vi "ArmControlManager.vi"(0 "Arm Rotate Manual Control":dbl, 1 "Arm Extend Manual Control":dbl, 2 "rotate sensor unit conversion (ticks/rad)":dbl, 3 "extend sensor unit coversion (ticks/in)":dbl, 4 "Arm Rotate Motion Profile":T1[](array[typedef]) {"Time (ms)" items=["TrajectoryDuration_0ms"=0, "TrajectoryDuration_5ms"=5, "TrajectoryDuration_10ms"=10, "TrajectoryDuration_20ms"=20, "TrajectoryDuration_30ms"=30, "TrajectoryDuration_40ms"=40, "TrajectoryDuration_50ms"=50, "TrajectoryDuration_100ms"=100]}, 5 "Arm Extend Motion Profile":T1[](array[typedef]) {"Time (ms)" items=["TrajectoryDuration_0ms"=0, "TrajectoryDuration_5ms"=5, "TrajectoryDuration_10ms"=10, "TrajectoryDuration_20ms"=20, "TrajectoryDuration_30ms"=30, "TrajectoryDuration_40ms"=40, "TrajectoryDuration_50ms"=50, "TrajectoryDuration_100ms"=100]}, 8 "Arm Extend Motor DevRef":T4={"DeviceStatus"={"status"=FALSE, "code"=0, "source"=""}, "Type"=enum."PWM", "PWM"={"PWM Channel"=enum."PWM 1", "DeadBand"={"Name"="", "maxPositivePwm"=0, "minPositivePwm"=0, "centerPwm"=0, "maxNegativePwm"=0, "minNegativePwm"=0, "angularRange"=0}}, "CAN"={"Device Number"=0, "SetOutput VI Ref"=variant(enum8{"Percent VBus", "Current", "Speed", "Position", "Voltage"} enum."Percent VBus"), "GetOutput VI Ref"=variant(refnum<k1> refnum), "Enable VI Ref"=variant(dbl 12.0), "Disable VI Ref"=variant(enum8{"Percent VBus", "Speed", "Position", "Slave", "Unchanged / Invalid", "Voltage Compensation", "Current", "Motion Profile"} enum."Percent VBus"), "Data"=variant}, "Invert"=FALSE, "DIO PWM"={"PWM \"Enable\" Channel"=enum."Invalid", "DIOChannel"=enum."Invalid", "PWM Rate"=0.0}}, 9 "New Motion Profile":bool, 10 "Arm Rotate Motor DevRef":T4={"DeviceStatus"={"status"=FALSE, "code"=0, "source"=""}, "Type"=enum."PWM", "PWM"={"PWM Channel"=enum."PWM 1", "DeadBand"={"Name"="", "maxPositivePwm"=0, "minPositivePwm"=0, "centerPwm"=0, "maxNegativePwm"=0, "minNegativePwm"=0, "angularRange"=0}}, "CAN"={"Device Number"=0, "SetOutput VI Ref"=variant(enum8{"Percent VBus", "Current", "Speed", "Position", "Voltage"} enum."Percent VBus"), "GetOutput VI Ref"=variant(refnum<k1> refnum), "Enable VI Ref"=variant(dbl 12.0), "Disable VI Ref"=variant(enum8{"Percent VBus", "Speed", "Position", "Slave", "Unchanged / Invalid", "Voltage Compensation", "Current", "Motion Profile"} enum."Percent VBus"), "Data"=variant}, "Invert"=FALSE, "DIO PWM"={"PWM \"Enable\" Channel"=enum."Invalid", "DIOChannel"=enum."Invalid", "PWM Rate"=0.0}}) -> (14 "Arm Control State":T3)   [LabVIEW 2017]
uses:
  General/MotionProfiling/TypeDefs/TrajectoryPoint.ctl
  <vilib>/Rock Robotics/WPI/ThirdParty/Phoenix-LabVIEW/Motor Controller/Controls/CTRE_Phoenix_MotorControl_TrajectoryPointTimeDur.ctl
  General/MotionProfiling/TypeDefs/MotionProfileControlState.ctl
  <vilib>/Rock Robotics/WPI/MotorControl/WPI_MotorControlDeviceRef.ctl
  <vilib>/Rock Robotics/WPI/MotorControl/WPI_MotorControlType.ctl
  <vilib>/Rock Robotics/SystemInterfaces/DIO/FPGA_DIOPWMChannel.ctl
  <vilib>/Rock Robotics/WPI/PWM/WPI_PWMDeadband.ctl
  <vilib>/Rock Robotics/SystemInterfaces/DIO/FPGA_DIOChannel.ctl
  <vilib>/Rock Robotics/WPI/DriverStation/WPI_DriverStationRobotMode2.ctl
  ArgosLib/Signal Processing/TypeDefs/EdgeDetector_Type.ctl
  <vilib>/Rock Robotics/WPI/ThirdParty/Phoenix-LabVIEW/Motor Controller/Controls/CTRE_Phoenix_MotorControl_ControlMode.ctl
  <vilib>/Rock Robotics/WPI/ThirdParty/Phoenix-LabVIEW/Motor Controller/Get/CTRE_Phoenix_MotorController_GetSelectedSensorData.vi
  <vilib>/Rock Robotics/WPI/ThirdParty/Phoenix-LabVIEW/Motor Controller/Get/CTRE_Phoenix_MotorController_GetClosedLoopData.vi
  <vilib>/Rock Robotics/WPI/ThirdParty/Phoenix-LabVIEW/Motor Controller/Get/CTRE_Phoenix_MotorController_GetVoltage.vi
  ArgosLib/ArgosLib.lvlib
panel:
  in  "Tab Control":enum32{"I/O", "Calibration", "Status"}(tab)
  in  "ExtendErrorThresh (in)":dbl=3.0
  in  "RotateErrorThresh (rad)":dbl=0.1745
  in  "ClearMotionProfile":bool
  in  "StallDetectTime(ms)":u32=200
  out "Max Extend Speed (Sensor Units per 100 ms)":i32
  out "Max Rotate Speed (Sensor Units per 100 ms)":i32
  in  "Reset Rotate Max":bool
  in  "Reset Extend Max":bool
  in  "Reset Extend Sensor":bool
  in  "Reset Rotate Sensor":bool
  in  "Extend Position (in)":dbl=-44.0
  in  "Rotate Position (rad)":dbl=1.57
  out "Rotate":T9
  out "Extension":T9
  out "Rotate":T10
  out "Extension":T10
  out "ExtendFaults":T11
  out "RotateFaults":T11
  out "Arm Tracking":cluster{dbl[], dbl[]}[](graph)
  out "ArmRotateV":dbl(graph)
  out "ArmExtensionV":dbl(graph)
  out "ArmExtension":T10(graph)
  out "ArmRotation":T10(graph)
  # "10 degrees or 3 inches\nerror for 200ms will\ncancel motion"
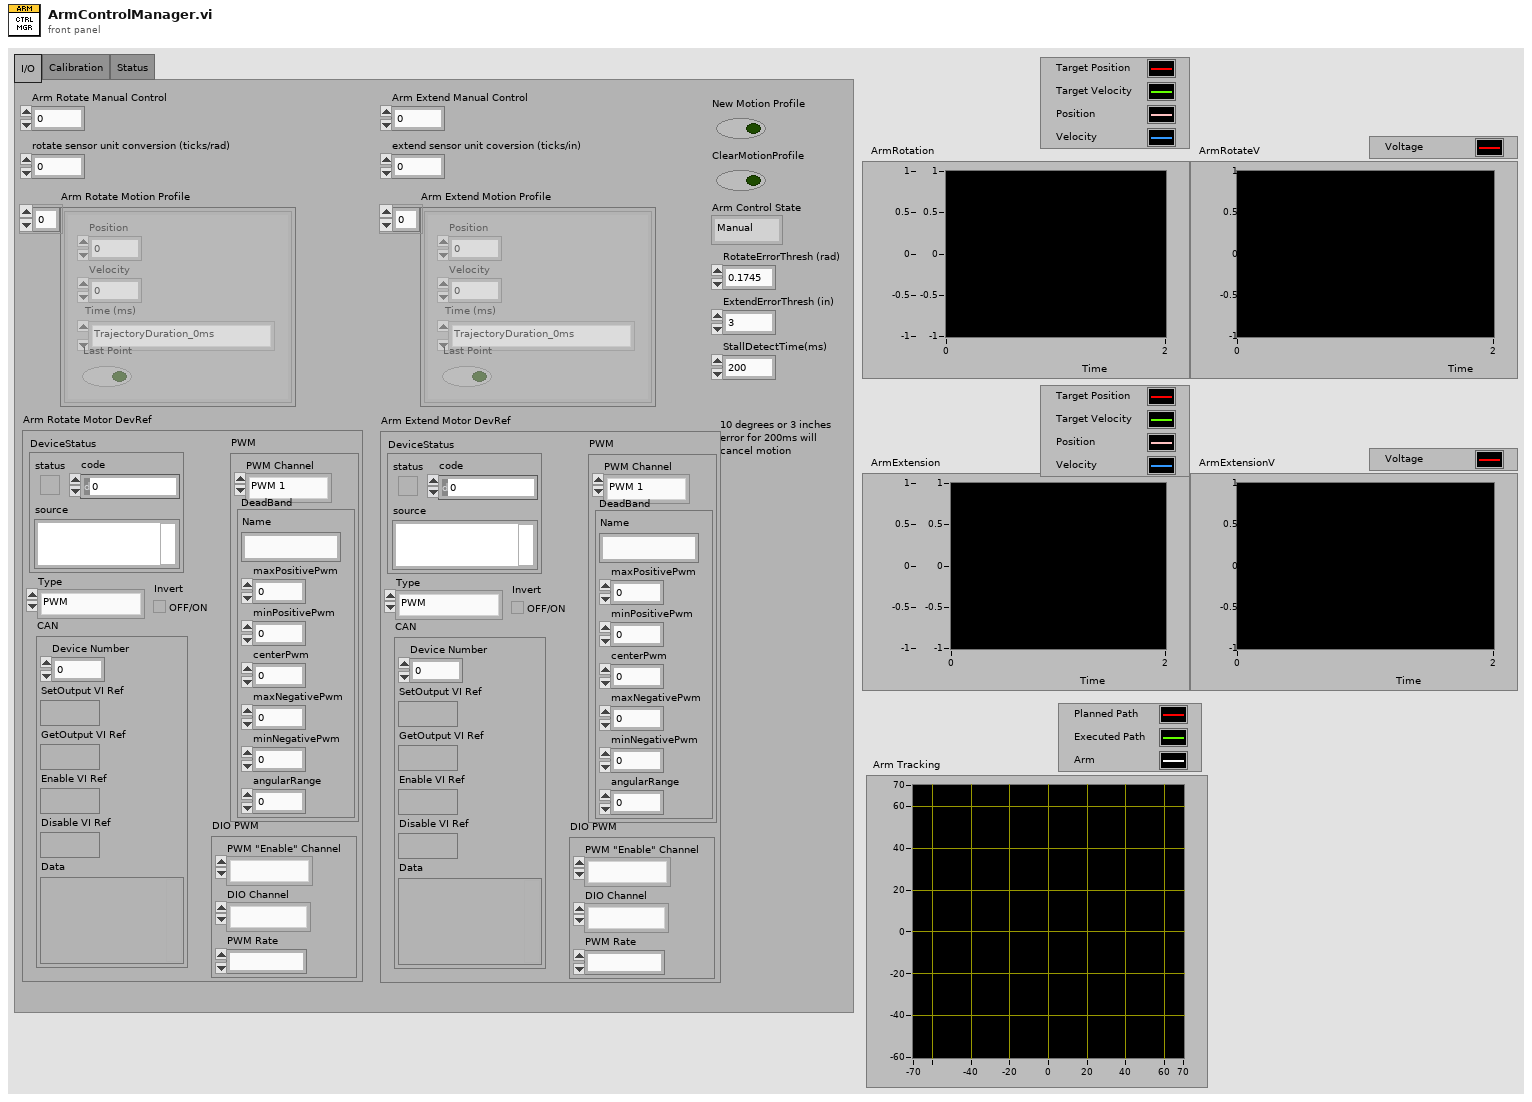
[diagram p1: front panel]
types:
  T1 = typedef "TrajectoryPoint.ctl" = cluster{"Position ":dbl, "Velocity ":dbl, "Time (ms)":T2, "Last Point":bool}
  T2 = typedef "CTRE_Phoenix_MotorControl_TrajectoryPointTimeDur.ctl" = i32
  T3 = typedef "MotionProfileControlState.ctl" = enum16{"Manual", "Auto_Idle", "Auto_Run"}
  T4 = typedef "WPI_MotorControlDeviceRef.ctl" = cluster{"DeviceStatus":errorcluster, "Type":T5, "PWM":cluster{"PWM Channel":T6, "DeadBand":T7}, "CAN":cluster{"Device Number":u8, "SetOutput VI Ref":variant, "GetOutput VI Ref":variant, "Enable VI Ref":variant, "Disable VI Ref":variant, "Data":variant}, "Invert":bool, "DIO PWM":cluster{"PWM \"Enable\" Channel":T6, "DIOChannel":T8, "PWM Rate":dbl}}
  T5 = typedef "WPI_MotorControlType.ctl" = enum16{"PWM", "CAN", "DIO PWM"}
  T6 = typedef "FPGA_DIOPWMChannel.ctl" = enum8{"PWM 0", "PWM 1", "PWM 2", "PWM 3", "PWM 4", "PWM 5", "PWM 6", "PWM 7", "PWM 8", "PWM 9", "PWM MXP 0", "PWM MXP 1", "PWM MXP 2", "PWM MXP 3", "PWM MXP 4", "PWM MXP 5", "PWM MXP 6", "PWM MXP 7", "PWM MXP 8", "PWM MXP 9", "Invalid"}
  T7 = typedef "WPI_PWMDeadband.ctl" = cluster{"Name":string, "maxPositivePwm":i32, "minPositivePwm":i32, "centerPwm":i32, "maxNegativePwm":i32, "minNegativePwm":i32, "angularRange":u16}
  T8 = typedef "FPGA_DIOChannel.ctl" = enum8{"DIO 0", "DIO 1", "DIO 2", "DIO 3", "DIO 4", "DIO 5", "DIO 6", "DIO 7", "DIO 8", "DIO 9", "DIO MXP 0", "DIO MXP 1", "DIO MXP 2", "DIO MXP 3", "DIO MXP 4", "DIO MXP 5", "DIO MXP 6", "DIO MXP 7", "DIO MXP 8", "DIO MXP 9", "DIO MXP 10", "DIO MXP 11", "DIO MXP 12", "DIO MXP 13", "DIO MXP 14", "DIO MXP 15", "SPI Port CS1", "SPI Port CS2", "SPI Port CS3", "SPI Port MISO", "SPI Port MOSI", "Invalid"}
  T9 = cluster{"Top Buffer Remaining":i32, "Top Buffer Count":i32, "Bottom Buffer Count":i32, "Has Underrun?":bool, "Is Underrun?":bool, "Active Point Valid?":bool, "Is Last?":bool, "Profile Slot Select 0":i32, "Output Enable":i32, "Time Duration (ms)":i32, "Profile Slot Select 1":i32}
  T10 = cluster{"Position (Sensor Units)":i32, "Velocity (Sensor Units per 100 ms)":i32, "Position (Raw Sensor Units)":i32, "Velocity (Raw Sensor Units per 100 ms)":i32}
  T11 = cluster{"Under Voltage":bool, "Forward Limit Switch":bool, "Reverse Limit Switch":bool, "Forward Soft Limit":bool, "Reverse Soft Limit":bool, "Hardware Failure":bool, "Reset During Enable":bool, "Sensor Overflow":bool, "Sensor Out of Phase":bool, "Hardware ESD Reset":bool, "Remote Loss of Signal":bool}
  T12 = typedef "WPI_DriverStationRobotMode2.ctl" = enum16{"Autonomous Disabled", "Autonomous Enabled", "Teleop Disabled", "Teleop Enabled", "Disconnected", "Finish", "Test Disabled", "Test Enabled", "Emergency Stopped"}
  T13 = typedef "ArgosLib.lvlib/EdgeDetector_Type.ctl" = enum16{"RisingEdge", "FallingEdge", "Both"}
  T14 = cluster{"Position (Sensor Units)":i32, "Velocity (Sensor Units per 100 ms)":i32, "Position (Raw Sensor Units)":i32, "Velocity (Raw Sensor Units per 100 ms)":i32}[]
  T15 = typedef "CTRE_Phoenix_MotorControl_ControlMode.ctl" = u16
  T16 = cluster{"Position (Sensor Units)":i32, "Velocity (Sensor Units per 100 ms)":i32, "Position (Raw Sensor Units)":i32, i32}
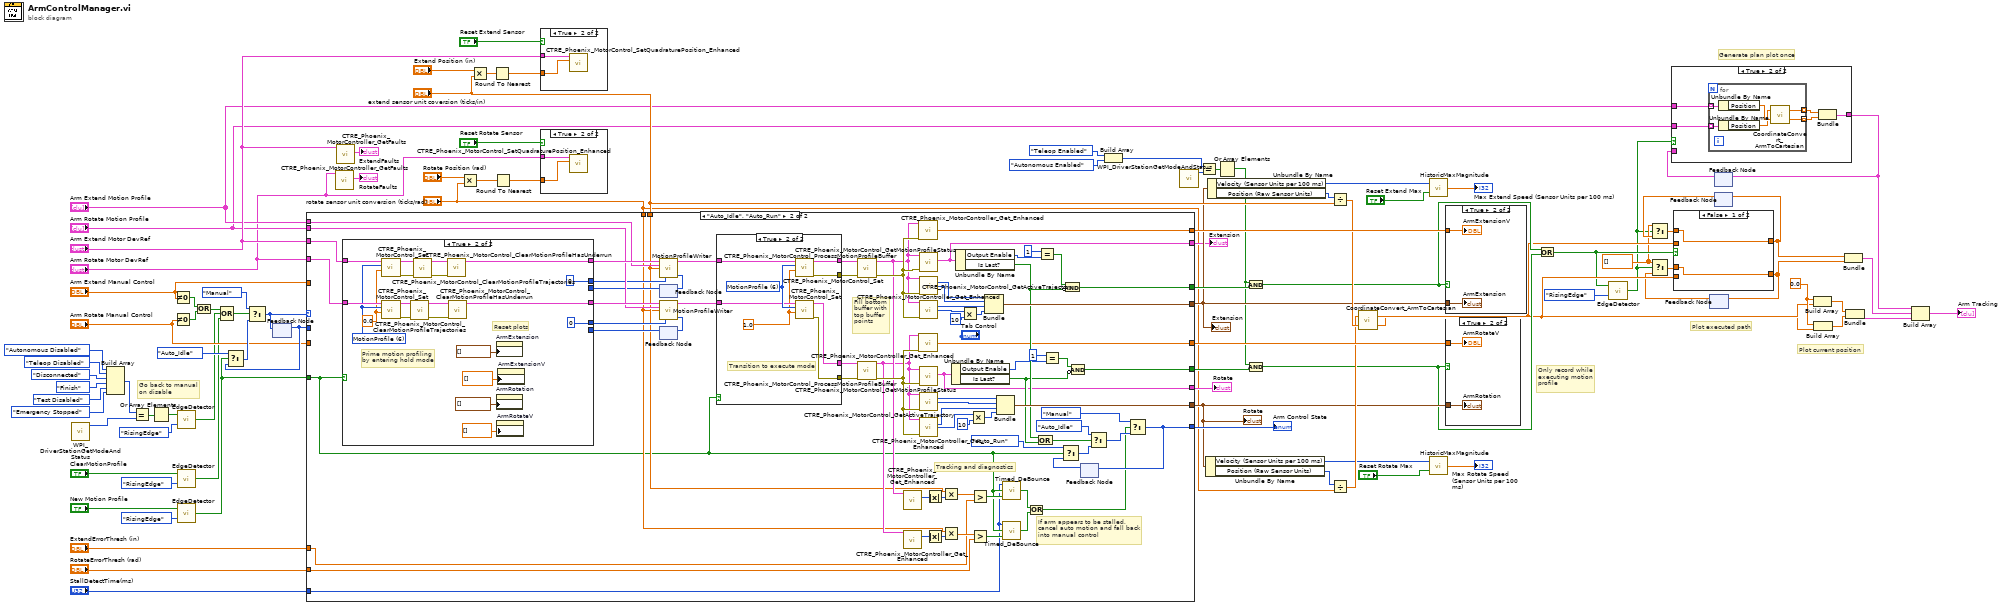
[diagram p0: block diagram]
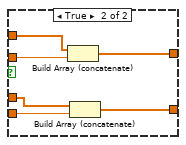
[diagram p3: hidden frame]
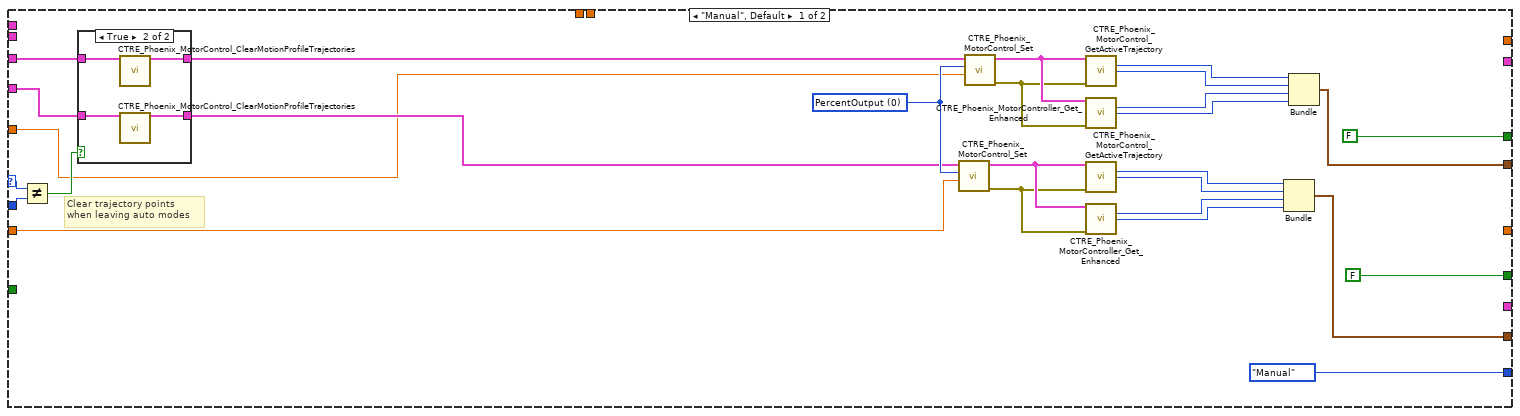
[diagram p8: hidden frame]
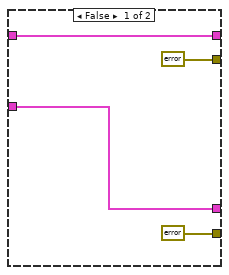
[diagram p10: hidden frame]
diagram:
  w16 = dbl[] [] ("t")
  w53 = 0.0 ("element")
  # "Plot current position"
  # "Plot executed path"
  # "Generate plan plot once"
  # "Go back to manual\non disable"
  # "Only record while\nexecuting motion\nprofile"
  n1 = call <vilib>:"WPI_DriverStationGetModeAndStatus.vi"() -> ("Robot Mode"=w45:T12)  [unwired: 10 in, 1 out]
  n2 = Build Array(WPI_DriverStationRobotMode2."Autonomous Disabled" ("Robot Mode"), WPI_DriverStationRobotMode2."Teleop Disabled" ("Robot Mode"), WPI_DriverStationRobotMode2."Disconnected" ("Robot Mode"), WPI_DriverStationRobotMode2."Finish" ("Robot Mode"), WPI_DriverStationRobotMode2."Test Disabled" ("Robot Mode"), WPI_DriverStationRobotMode2."Emergency Stopped" ("Robot Mode")) -> (w46:T12[])
  n3 = Equal?(x=w46, y=w45) -> (x = y?=w44:bool[])
  n4 = Or Array Elements(Boolean array=w44) -> (logical OR=w43:bool)
  n5 = Not Equal To 0?(x="Arm Extend Manual Control") -> (x != 0?=w95:bool)
  n6 = Not Equal To 0?(x="Arm Rotate Manual Control") -> (x != 0?=w94:bool)
  n7 = call "EdgeDetector.vi"("DetectorType"=EdgeDetector_Type."RisingEdge", "Input"=w43) -> ("Edge"=w40:bool)
  n8 = call "EdgeDetector.vi"("DetectorType"=EdgeDetector_Type."RisingEdge", "Input"="ClearMotionProfile") -> ("Edge"=w41:bool)
  n9 = call "EdgeDetector.vi"("DetectorType"=EdgeDetector_Type."RisingEdge", "Input"="New Motion Profile") -> ("Edge"=w87:bool)
  n10 = Or(x=w95, y=w94) -> (x .or. y?=w72:bool)
  n11 = Compound Arithmetic op=OR(w72, w40, w41) -> (w73:bool)
  n12 = feedback #1() -> (w91:T3)  [unwired: 1 in]
  n13 = Select(t=MotionProfileControlState."Auto_Idle", s=w87, f=w91) -> (s? t:f=w92:T3)
  n14 = Select(t=MotionProfileControlState."Manual" ("Arm Control State"), s=w73, f=w92) -> (s? t:f=w39:T3)
  n15 = feedback-in #1(w39) -> ()
  n16 = case shown="\"Auto_Idle\", \"Auto_Run\"" w39 {
    selector: w39 -> [w120 _]
    tunnel: "Arm Extend Motor DevRef" -> [w117 w203]
    tunnel: "Arm Rotate Motor DevRef" -> [w115 w202]
    tunnel: "Arm Extend Manual Control" -> [w96 _]
    tunnel: "Arm Rotate Manual Control" -> [w121 _]
    tunnel: w91 -> [w119 _]
    tunnel: w87 -> [_ w136]
    tunnel: "Arm Extend Motion Profile" -> [_ w189]
    tunnel: "Arm Rotate Motion Profile" -> [_ w188]
    tunnel: [MotionProfileControlState."Manual" ("Arm Control State") w132] -> w86
    tunnel: [w112 w193] -> w55
    tunnel: [w99 w192] -> w54
    tunnel: [FALSE w173] -> w76
    tunnel: [FALSE w169] -> w79
    tunnel: [_ w160] -> w75
    tunnel: [_ w159] -> w74
    tunnel: "extend sensor unit coversion (ticks/in)" -> [_ w147]
    tunnel: "rotate sensor unit conversion (ticks/rad)" -> [_ w143]
    tunnel: [_ w154] -> w32
    tunnel: [_ w153] -> w31
    tunnel: "ExtendErrorThresh (in)" -> [_ w139]
    tunnel: "RotateErrorThresh (rad)" -> [_ w140]
    tunnel: "StallDetectTime(ms)" -> [_ w135]
    frame "Manual", Default {
      w122 = T15 0 items=["PercentOutput"=0, "Position"=1, "Velocity"=2, "Current"=3, "Follower"=5, "MotionProfile"=6, "MotionMagic"=7, "MotionMagicArc"=8, "MotionProfileArc"=10, "Disabled"=15] ("Control Mode")
      # "Clear trajectory points\nwhen leaving auto modes"
      n17 = Not Equal?(x=w120, y=w119) -> (x != y?=w118:bool)
      n18 = case shown="True" w118 {
        tunnel: w117 -> [w124 w128]
        tunnel: [w124 w127] -> w116
        tunnel: w115 -> [w123 w126]
        tunnel: [w123 w125] -> w114
        frame False {
        }
        frame True {
          n19 = call <vilib>:"CTRE_Phoenix_MotorControl_ClearMotionProfileTrajectories.vi"("PhoenixMotorControlDevRef"=w128) -> ("PhoenixMotorControlDevRef"=w127:T4)  [unwired: 13 in, 1 out]
          n20 = call <vilib>:"CTRE_Phoenix_MotorControl_ClearMotionProfileTrajectories.vi"("PhoenixMotorControlDevRef"=w126) -> ("PhoenixMotorControlDevRef"=w125:T4)  [unwired: 13 in, 1 out]
        }
      }
      n21 = call <vilib>:"CTRE_Phoenix_MotorControl_Set.vi"("Output"=w121, "Control Mode"=w122, "PhoenixMotorControlDevRef"=w114) -> ("error out"=w104:errorcluster, "PhoenixMotorControlDevRef"=w105:T4)  [unwired: 7 in]
      n22 = call <vilib>:"CTRE_Phoenix_MotorControl_Set.vi"("Output"=w96, "Control Mode"=w122, "PhoenixMotorControlDevRef"=w116) -> ("error out"=w110:errorcluster, "PhoenixMotorControlDevRef"=w111:T4)  [unwired: 7 in]
      n23 = call <vilib>:"CTRE_Phoenix_MotorControl_GetActiveTrajectory.vi"("PhoenixMotorControlDevRef"=w111, "error in"=w110) -> ("Position (Sensor Units)"=w109:i32, "Velocity (Sensor Units per 100 ms)"=w108:i32)  [unwired: 9 in, 3 out]
      n24 = call-poly <vilib>:"CTRE_Phoenix_MotorController_Get_Enhanced.vi"("PhoenixMotorControlDevRef"=w111, "error in"=w110) -> ("Position (Raw Sensor Units)"=w107:i32, "Velocity (Raw Sensor Units per 100 ms)"=w106:i32)  [unwired: 10 in, 2 out]
      n25 = call <vilib>:"CTRE_Phoenix_MotorControl_GetActiveTrajectory.vi"("PhoenixMotorControlDevRef"=w105, "error in"=w104) -> ("Position (Sensor Units)"=w103:i32, "Velocity (Sensor Units per 100 ms)"=w102:i32)  [unwired: 9 in, 3 out]
      n26 = call-poly <vilib>:"CTRE_Phoenix_MotorController_Get_Enhanced.vi"("PhoenixMotorControlDevRef"=w105, "error in"=w104) -> ("Position (Raw Sensor Units)"=w101:i32, "Velocity (Raw Sensor Units per 100 ms)"=w100:i32)  [unwired: 10 in, 2 out]
      n27 = Bundle("Position (Sensor Units)"=w103, "Velocity (Sensor Units per 100 ms)"=w102, "Position (Raw Sensor Units)"=w101, "Velocity (Raw Sensor Units per 100 ms)"=w100) -> (w99:T10)  [unwired: 1 in]
      n28 = Bundle("Position (Sensor Units)"=w109, "Velocity (Sensor Units per 100 ms)"=w108, "Position (Raw Sensor Units)"=w107, "Velocity (Raw Sensor Units per 100 ms)"=w106) -> (w112:T10)  [unwired: 1 in]
    }
    frame "Auto_Idle", "Auto_Run" {
      # "If arm appears to be stalled,\ncancel auto motion and fall back\ninto manual control"
      # "Tracking and diagnostics"
      # "Fill bottom\nbuffer with\ntop buffer\npoints"
      n29 = feedback #2() -> (w182:i32)  [unwired: 1 in]
      n30 = feedback #3() -> (w184:i32)  [unwired: 1 in]
      n31 = case shown="True" w136 {
        tunnel: w203 -> [w219 w227]
        tunnel: w202 -> [w218 w224]
        tunnel: [w219 w231] -> w190
        tunnel: [w218 w230] -> w191
        tunnel: [w216 0] -> w187
        tunnel: [w217 0] -> w186
        tunnel: w184 -> [w217 _]
        tunnel: w182 -> [w216 _]
        frame False {
        }
        frame True {
          w222 = 0.0 ("Output")
          w223 = T15 6 items=["PercentOutput"=0, "Position"=1, "Velocity"=2, "Current"=3, "Follower"=5, "MotionProfile"=6, "MotionMagic"=7, "MotionMagicArc"=8, "MotionProfileArc"=10, "Disabled"=15] ("Control Mode")
          # "Prime motion profiling\nby entering hold mode"
          # "Reset plots"
          n32 = call <vilib>:"CTRE_Phoenix_MotorControl_Set.vi"("Output"=w222, "Control Mode"=w223, "PhoenixMotorControlDevRef"=w227) -> ("error out"=w229:errorcluster, "PhoenixMotorControlDevRef"=w228:T4)  [unwired: 7 in]
          n33 = call <vilib>:"CTRE_Phoenix_MotorControl_Set.vi"("Output"=w222, "Control Mode"=w223, "PhoenixMotorControlDevRef"=w224) -> ("error out"=w226:errorcluster, "PhoenixMotorControlDevRef"=w225:T4)  [unwired: 7 in]
          n34 = call <vilib>:"CTRE_Phoenix_MotorControl_ClearMotionProfileTrajectories.vi"("PhoenixMotorControlDevRef"=w225, "error in"=w226) -> ("PhoenixMotorControlDevRef"=w235:T4, "error out"=w234:errorcluster)  [unwired: 12 in]
          n35 = call <vilib>:"CTRE_Phoenix_MotorControl_ClearMotionProfileTrajectories.vi"("PhoenixMotorControlDevRef"=w228, "error in"=w229) -> ("PhoenixMotorControlDevRef"=w233:T4, "error out"=w232:errorcluster)  [unwired: 12 in]
          n36 = call <vilib>:"CTRE_Phoenix_MotorControl_ClearMotionProfileHasUnderrun.vi"("error in"=w232, "PhoenixMotorControlDevRef"=w233) -> ("PhoenixMotorControlDevRef"=w231:T4)  [unwired: 8 in, 1 out]
          n37 = call <vilib>:"CTRE_Phoenix_MotorControl_ClearMotionProfileHasUnderrun.vi"("error in"=w234, "PhoenixMotorControlDevRef"=w235) -> ("PhoenixMotorControlDevRef"=w230:T4)  [unwired: 8 in, 1 out]
          n38 = property on="ArmExtension" class="WFChart (strict)"("History Data"=T14 []) -> ()  [unwired: 2 in, 2 out]
          n39 = property on="ArmRotation" class="WFChart (strict)"("History Data"=T14 []) -> ()  [unwired: 2 in, 2 out]
          n40 = property on="ArmRotateV" class="WFChart (strict)"("History Data"=dbl[] []) -> ()  [unwired: 2 in, 2 out]
          n41 = property on="ArmExtensionV" class="WFChart (strict)"("History Data"=dbl[] []) -> ()  [unwired: 2 in, 2 out]
        }
      }
      n42 = call "MotionProfileWriter.vi"("PhoenixMotorControlDevRef"=w190, "Trajectory Points"=w189, "Sensor unit conversion"=w147, "startIndex"=w187) -> ("PhoenixMotorControlDevRef Out"=w181:T4, "endIndex"=w183:i32)  [unwired: 10 in]
      n43 = feedback-in #2(w183) -> ()
      n44 = call "MotionProfileWriter.vi"("PhoenixMotorControlDevRef"=w191, "Trajectory Points"=w188, "Sensor unit conversion"=w143, "startIndex"=w186) -> ("PhoenixMotorControlDevRef Out"=w179:T4, "endIndex"=w185:i32)  [unwired: 10 in]
      n45 = feedback-in #3(w185) -> ()
      n46 = case shown="True" w136 {
        tunnel: w181 -> [w207 w214]
        tunnel: [w207 w213] -> w180
        tunnel: w179 -> [w206 w212]
        tunnel: [w206 w211] -> w178
        tunnel: [errorcluster {"status"=FALSE, "code"=0, "source"=""} ("error out") w209] -> w152
        tunnel: [errorcluster {"status"=FALSE, "code"=0, "source"=""} ("error out") w208] -> w151
        frame False {
        }
        frame True {
          w210 = 1.0 ("Output")
          w215 = T15 6 items=["PercentOutput"=0, "Position"=1, "Velocity"=2, "Current"=3, "Follower"=5, "MotionProfile"=6, "MotionMagic"=7, "MotionMagicArc"=8, "MotionProfileArc"=10, "Disabled"=15] ("Control Mode")
          # "Transition to execute mode"
          n47 = call <vilib>:"CTRE_Phoenix_MotorControl_Set.vi"("Output"=w210, "Control Mode"=w215, "PhoenixMotorControlDevRef"=w214) -> ("error out"=w209:errorcluster, "PhoenixMotorControlDevRef"=w213:T4)  [unwired: 7 in]
          n48 = call <vilib>:"CTRE_Phoenix_MotorControl_Set.vi"("Output"=w210, "Control Mode"=w215, "PhoenixMotorControlDevRef"=w212) -> ("error out"=w208:errorcluster, "PhoenixMotorControlDevRef"=w211:T4)  [unwired: 7 in]
        }
      }
      n49 = call <vilib>:"CTRE_Phoenix_MotorControl_ProcessMotionProfileBuffer.vi"("PhoenixMotorControlDevRef"=w180, "error in"=w152) -> ("PhoenixMotorControlDevRef"=w150:T4, "error out"=w162:errorcluster)  [unwired: 12 in]
      n50 = call <vilib>:"CTRE_Phoenix_MotorControl_ProcessMotionProfileBuffer.vi"("PhoenixMotorControlDevRef"=w178, "error in"=w151) -> ("PhoenixMotorControlDevRef"=w149:T4, "error out"=w161:errorcluster)  [unwired: 12 in]
      n51 = call-poly <vilib>:"CTRE_Phoenix_MotorController_Get_Enhanced.vi"("PhoenixMotorControlDevRef"=w150) -> ("Closed-loop Error"=w148:i32)  [unwired: 9 in, 5 out]
      n52 = call-poly <vilib>:"CTRE_Phoenix_MotorController_Get_Enhanced.vi"("PhoenixMotorControlDevRef"=w149) -> ("Closed-loop Error"=w144:i32)  [unwired: 9 in, 5 out]
      n53 = call-poly <vilib>:"CTRE_Phoenix_MotorController_Get_Enhanced.vi"("PhoenixMotorControlDevRef"=w150, "error in"=w162) -> ("Output Voltage"=w159:dbl)  [unwired: 9 in, 4 out]
      n54 = call-poly <vilib>:"CTRE_Phoenix_MotorController_Get_Enhanced.vi"("PhoenixMotorControlDevRef"=w149, "error in"=w161) -> ("Output Voltage"=w160:dbl)  [unwired: 9 in, 4 out]
      n55 = call <vilib>:"CTRE_Phoenix_MotorControl_GetMotionProfileStatus.vi"("error in"=w162, "PhoenixMotorControlDevRef"=w150) -> ("Motion Profile Status"=w153:T9)  [unwired: 7 in, 2 out]
      n56 = call <vilib>:"CTRE_Phoenix_MotorControl_GetActiveTrajectory.vi"("PhoenixMotorControlDevRef"=w150, "error in"=w162) -> ("Position (Sensor Units)"=w199:i32, "Velocity (Sensor Units per 100 ms)"=w198:i32)  [unwired: 9 in, 3 out]
      n57 = call-poly <vilib>:"CTRE_Phoenix_MotorController_Get_Enhanced.vi"("PhoenixMotorControlDevRef"=w150, "error in"=w162) -> ("Position (Raw Sensor Units)"=w197:i32, "Velocity (Raw Sensor Units per 100 ms)"=w164:i32)  [unwired: 10 in, 2 out]
      n58 = call <vilib>:"CTRE_Phoenix_MotorControl_GetMotionProfileStatus.vi"("error in"=w161, "PhoenixMotorControlDevRef"=w149) -> ("Motion Profile Status"=w154:T9)  [unwired: 7 in, 2 out]
      n59 = call <vilib>:"CTRE_Phoenix_MotorControl_GetActiveTrajectory.vi"("PhoenixMotorControlDevRef"=w149, "error in"=w161) -> ("Position (Sensor Units)"=w196:i32, "Velocity (Sensor Units per 100 ms)"=w195:i32)  [unwired: 9 in, 3 out]
      n60 = call-poly <vilib>:"CTRE_Phoenix_MotorController_Get_Enhanced.vi"("PhoenixMotorControlDevRef"=w149, "error in"=w161) -> ("Position (Raw Sensor Units)"=w194:i32, "Velocity (Raw Sensor Units per 100 ms)"=w167:i32)  [unwired: 10 in, 2 out]
      n61 = Absolute Value(x=w148) -> (abs(x)=w146:i32)
      n62 = Absolute Value(x=w144) -> (abs(x)=w145:i32)
      n63 = Multiply(x=w147, y=w146) -> (x*y=w142:dbl)
      n64 = Multiply(x=w143, y=w145) -> (x*y=w141:dbl)
      n65 = Unbundle By Name(w154) -> ("Output Enable"=w170:i32, "Is Last?"=w158:bool)
      n66 = Unbundle By Name(w153) -> ("Output Enable"=w177:i32, "Is Last?"=w174:bool)
      n67 = Multiply(x=w164, y=10) -> (x*y=w165:i32)
      n68 = Multiply(x=w167, y=10) -> (x*y=w168:i32)
      n69 = Greater?(x=w142, y=w139) -> (0:w138:bool)
      n70 = Greater?(x=w141, y=w140) -> (0:w137:bool)
      n71 = Bundle("Position (Sensor Units)"=w199, "Velocity (Sensor Units per 100 ms)"=w198, "Position (Raw Sensor Units)"=w197, w165) -> (w193:T16)  [unwired: 1 in]
      n72 = Bundle("Position (Sensor Units)"=w196, "Velocity (Sensor Units per 100 ms)"=w195, "Position (Raw Sensor Units)"=w194, w168) -> (w192:T16)  [unwired: 1 in]
      n73 = call "Timed_DeBounce.vi"("Input"=w138, "Reset"=w136, "Hold Time(ms)"=w135) -> ("Output"=w134:bool)
      n74 = call "Timed_DeBounce.vi"("Input"=w137, "Reset"=w136, "Hold Time(ms)"=w135) -> ("Output"=w133:bool)
      n75 = Or(x=w134, y=w133) -> (x .or. y?=w129:bool)
      n76 = Equal?(x=1, y=w177) -> (x = y?=w175:bool)
      n77 = Compound Arithmetic op=OR(w174, w158) -> (w201:bool)
      n78 = Equal?(x=1, y=w170) -> (x = y?=w172:bool)
      n79 = Compound Arithmetic op=AND(w175, invert w174) -> (w173:bool)
      n80 = Compound Arithmetic op=AND(w172, invert w158) -> (w169:bool)
      n81 = feedback #4() -> (w155:T3)  [unwired: 1 in]
      n82 = Select(t=MotionProfileControlState."Auto_Run" ("Arm Control State"), s=w136, f=w155) -> (s? t:f=w156:T3)
      n83 = Select(t=MotionProfileControlState."Auto_Idle" ("Arm Control State"), s=w201, f=w156) -> (s? t:f=w131:T3)
      n84 = Select(t=MotionProfileControlState."Manual", s=w129, f=w131) -> (s? t:f=w132:T3)
      n85 = feedback-in #4(w132) -> ()
    }
  }
  "Arm Control State" <- w86
  "Extension" <- w55
  "Rotate" <- w54
  "Rotate" <- w32
  "Extension" <- w31
  n86 = call <vilib>:"CTRE_Phoenix_MotorController_GetFaults.vi"("PhoenixMotorControlDevRef"="Arm Rotate Motor DevRef") -> ("Faults"=→"RotateFaults":T11)  [unwired: 8 in, 2 out]
  n87 = call <vilib>:"CTRE_Phoenix_MotorController_GetFaults.vi"("PhoenixMotorControlDevRef"="Arm Extend Motor DevRef") -> ("Faults"=→"ExtendFaults":T11)  [unwired: 8 in, 2 out]
  n88 = Multiply(x="Rotate Position (rad)", y="rotate sensor unit conversion (ticks/rad)") -> (x*y=w57:dbl)
  n89 = Multiply(x="Extend Position (in)", y="extend sensor unit coversion (ticks/in)") -> (x*y=w60:dbl)
  n90 = Round To Nearest(number=w60) -> (nearest integer value=w59:dbl)
  n91 = Round To Nearest(number=w57) -> (nearest integer value=w56:dbl)
  n92 = case shown="True" "Reset Extend Sensor" {
    tunnel: "Arm Extend Motor DevRef" -> [_ w241]
    tunnel: w59 -> [_ w240]
    frame False {
    }
    frame True {
      n93 = call <vilib>:"CTRE_Phoenix_MotorControl_SetQuadraturePosition_Enhanced.vi"("New Position"=w240, "PhoenixMotorControlDevRef"=w241) -> ()  [unwired: 8 in, 2 out]
    }
  }
  n94 = case shown="True" "Reset Rotate Sensor" {
    tunnel: "Arm Rotate Motor DevRef" -> [_ w243]
    tunnel: w56 -> [_ w242]
    frame False {
    }
    frame True {
      n95 = call <vilib>:"CTRE_Phoenix_MotorControl_SetQuadraturePosition_Enhanced.vi"("New Position"=w242, "PhoenixMotorControlDevRef"=w243) -> ()  [unwired: 8 in, 2 out]
    }
  }
  n96 = Build Array(WPI_DriverStationRobotMode2."Teleop Enabled" ("Robot Mode"), WPI_DriverStationRobotMode2."Autonomous Enabled" ("Robot Mode")) -> (w5:T12[])
  n97 = call <vilib>:"WPI_DriverStationGetModeAndStatus.vi"() -> ("Robot Mode"=w9:T12)  [unwired: 10 in, 1 out]
  n98 = Equal?(x=w5, y=w9) -> (x = y?=w8:bool[])
  n99 = Unbundle By Name(w54) -> ("Velocity (Sensor Units per 100 ms)"=w35:i32, "Position (Raw Sensor Units)"=w69:i32)
  n100 = Unbundle By Name(w55) -> ("Velocity (Sensor Units per 100 ms)"=w38:i32, "Position (Raw Sensor Units)"=w70:i32)
  n101 = Or Array Elements(Boolean array=w8) -> (logical OR=w4:bool)
  n102 = And(x=w4, y=w76) -> (x .and. y?=w29:bool)
  n103 = And(x=w4, y=w79) -> (x .and. y?=w28:bool)
  n104 = Divide(x=w70, y="extend sensor unit coversion (ticks/in)") -> (x/y=w68:dbl)
  n105 = Divide(x=w69, y="rotate sensor unit conversion (ticks/rad)") -> (x/y=w67:dbl)
  n106 = call "CoordinateConvert_ArmToCartesian.vi"("Radius (in)"=w68, "Angle (rad)"=w67) -> ("Y (in)"=w26:dbl, "X (in)"=w27:dbl)
  n107 = call "HistoricMaxMagnitude.vi"("Reset"="Reset Extend Max", "Value"=w38) -> ("Max"=→"Max Extend Speed (Sensor Units per 100 ms)":dbl)
  n108 = call "HistoricMaxMagnitude.vi"("Reset"="Reset Rotate Max", "Value"=w35) -> ("Max"=→"Max Rotate Speed (Sensor Units per 100 ms)":dbl)
  n109 = case shown="True" w29 {
    tunnel: w55 -> [_ w245]
    tunnel: w74 -> [_ w244]
    frame False {
    }
    frame True {
      "ArmExtension" <- w245
      "ArmExtensionV" <- w244
    }
  }
  n110 = case shown="True" w28 {
    tunnel: w54 -> [_ w247]
    tunnel: w75 -> [_ w246]
    frame False {
    }
    frame True {
      "ArmRotation" <- w247
      "ArmRotateV" <- w246
    }
  }
  n111 = Or(x=w29, y=w28) -> (x .or. y?=w23:bool)
  n112 = call "EdgeDetector.vi"("DetectorType"=EdgeDetector_Type."RisingEdge", "Input"=w23) -> ("Edge"=w10:bool)
  n113 = feedback #5() -> (w21:dbl[])  [unwired: 1 in]
  n114 = Select(t=w16, s=w10, f=w21) -> (s? t:f=w20:dbl[])
  n115 = feedback #6() -> (w12:cluster{dbl[], dbl[]})  [unwired: 1 in]
  n116 = case shown="True" w10 {
    tunnel: "Arm Extend Motion Profile" -> [_ w253]
    tunnel: "Arm Rotate Motion Profile" -> [_ w252]
    tunnel: [w248 w249] -> w13
    tunnel: w12 -> [w248 _]
    frame False {
    }
    frame True {
      n117 = for {
        tunnel: w253 -> [w259] mode=indexing
        tunnel: w252 -> [w258] mode=indexing
        tunnel: [w255] -> w251 mode=indexing
        tunnel: [w254] -> w250 mode=indexing
        n118 = Unbundle By Name(w259) -> ("Position"=w257:dbl)
        n119 = Unbundle By Name(w258) -> ("Position"=w256:dbl)
        n120 = call "CoordinateConvert_ArmToCartesian.vi"("Radius (in)"=w257, "Angle (rad)"=w256) -> ("Y (in)"=w254:dbl, "X (in)"=w255:dbl)
      }
      n121 = Bundle(w251, w250) -> (w249:cluster{dbl[], dbl[]})  [unwired: 1 in]
    }
  }
  n122 = feedback-in #6(w13) -> ()
  n123 = feedback #7() -> (w17:dbl[])  [unwired: 1 in]
  n124 = Select(t=w16, s=w10, f=w17) -> (s? t:f=w19:dbl[])
  n125 = case shown="False" w23 {
    tunnel: w27 -> [_ w267]
    tunnel: w26 -> [_ w266]
    tunnel: [w260 w265] -> w24
    tunnel: [w261 w264] -> w18
    tunnel: w20 -> [w260 w263]
    tunnel: w19 -> [w261 w262]
    frame False {
    }
    frame True {
      n126 = Build Array (concatenate)(w262, w267) -> (w264:dbl[])
      n127 = Build Array (concatenate)(w263, w266) -> (w265:dbl[])
    }
  }
  n128 = feedback-in #5(w24) -> ()
  n129 = feedback-in #7(w18) -> ()
  n130 = Build Array(w53, w27) -> (w66:dbl[])
  n131 = Build Array(w53, w26) -> (w65:dbl[])
  n132 = Bundle("t"=w18, "t"=w24) -> (w25:cluster{"t":dbl[], "t":dbl[]})  [unwired: 1 in]
  n133 = Bundle(w66, w65) -> (w64:cluster{dbl[], dbl[]})  [unwired: 1 in]
  n134 = Build Array(w13, w25, w64) -> (→"Arm Tracking":cluster{"t":dbl[], "t":dbl[]}[])
